vi "set constant value.vi"(7 "control name":string, 8 "error in":errorcluster, 9 "data to set":variant, 10 "vi path":path, 11 "application in":refnum<vi>) -> (0 "error out":errorcluster)   [LabVIEW 2014, in "SequencerActionScript.lvclass"]
doc: "NI Tag Bus Module Framework 1.0.2.36\nNI Systems Engineering"
uses:
  SequencerActionScript.lvclass
  <vilib>/Utility/traverseref.llb/TRef TravTarget.ctl
  <vilib>/Utility/traverseref.llb/VI Scripting - Traverse.lvlib
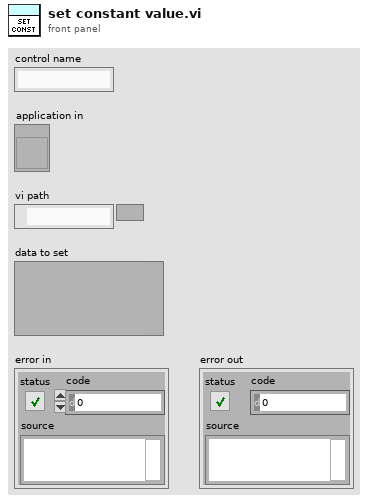
[diagram p1: front panel]
types:
  T1 = typedef "TRef TravTarget.ctl" = enum16{"FP", "BD", "Other"}
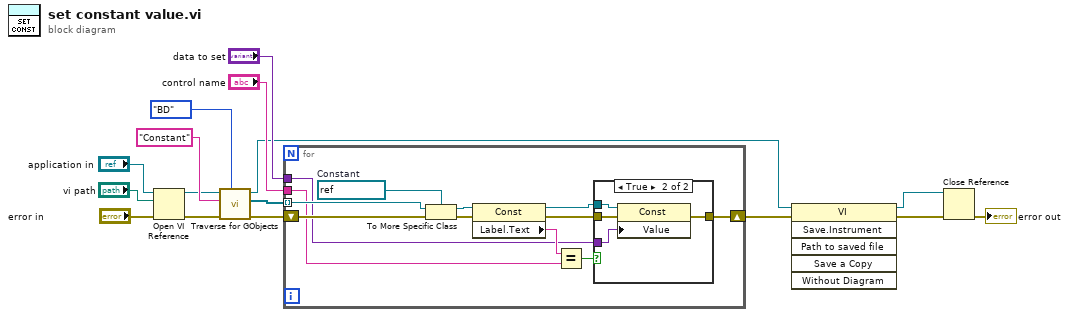
[diagram p0: block diagram]
diagram:
  n1 = Open VI Reference(application reference (local)="application in", vi path="vi path", error in (no error)="error in") -> (vi reference=w8:refnum<vi>, error out=w7:errorcluster)  [unwired: 3 in]
  n2 = call <vilib>:"Traverse for GObjects.vi"("Traverse Target"=TRef_TravTarget."BD", "error in (no error)"=w7, "Class Name"="Constant", "VI Refnum"=w8) -> ("error out"=w11:errorcluster, "References"=w12:refnum<vi>[], "dup VI Refnum"=w2:refnum<vi>)  [unwired: 4 in, 1 out]
  n3 = for {
    shift-right: [w21] -> w13
    shift-left: w11 -> [w28]
    tunnel: w12 -> [w27] mode=indexing
    tunnel: "control name" -> [w18]
    tunnel: "data to set" -> [w17]
    w26 = refnum<vi> refnum  # Constant
    n4 = To More Specific Class(target class=w26, reference=w27, error in=w28) -> (specific class reference=w25:refnum<vi>, error out=w24:errorcluster)
    n5 = property class="Const"(reference=w25, error in=w24) -> (reference out=w19:refnum<vi>, error out=w20:errorcluster, "Label.Text"=w23:string)
    n6 = Equal?(x=w23, y=w18) -> (x = y?=w22:bool)
    n7 = case shown="True" w22 {
      tunnel: [w29 w31] -> w21
      tunnel: w20 -> [w29 w33]
      tunnel: w19 -> [_ w32]
      tunnel: w17 -> [_ w30]
      frame False {
      }
      frame True {
        n8 = property class="Const"(reference=w32, error in=w33, "Value"=w30) -> (error out=w31:errorcluster)  [unwired: 1 out]
      }
    }
  }
  n9 = invoke class="VI" method="Save.Instrument"(reference=w2, error in=w13) -> (reference out=w1:refnum<vi>, error out=w3:errorcluster)  [unwired: 4 in, 4 out]
  n10 = Close Reference(reference=w1, error in (no error)=w3) -> (error out=→"error out":errorcluster)
